vi "Pump.vi"(2 "error in (no error)":errorcluster, 3 "Pump Frequency":i32=100, 4 "Pump Cycles":i32, 5 "LINX Resource":T1={"IO"=enum."Remote", "Interface"=enum."Serial", "LINX Device Config"={"Interface"=enum."Serial", "COM Port"="COM13", "TCP Configuration"={"IP Address"="", "Port"=0}, "Device Family"=1, "Device ID"=1, "Device Name"="myRIO-1900", "TCP Ref"=refnum, "Channels"={"DI"=[0, 1, 2, 3, 4, 5, 6, 7, 8, 9, 10, 11, 12, 13, 14, 15, 16, 17, 18, 19, 20, 21, 22, 23, 24, 25, 26, 27, 28, 29, 30, 31, 32, 33, 34, 35, 36, 37, 38, 39, 40, 41, 42, 43, 44, 45, 46], "DO"=[0, 1, 2, 3, 4, 5, 6, 7, 8, 9, 10, 11, 12, 13, 14, 15, 16, 17, 18, 19, 20, 21, 22, 23, 24, 25, 26, 27, 28, 29, 30, 31, 32, 33, 34, 35, 36, 37, 38, 39, 40, 41, 42, 43, 44, 45, 46], "AI"=[0, 1, 2, 3, 4, 5, 6, 7, 8, 9, 10, 11], "AO"=[], "PWM"=[3, 5, 6, 9, 10], "QE"=[], "UART"=[0, 1], "I2C 2"=[0], "SPI"=[0], "CAN"=[], "Servo"=[], "AI Ref (V)"=0.0, "AI Resolution (Bits)"=0, "AO Ref (V)"=0.0, "AO Resolution (Bits)"=0}}}) -> (0 "error out":errorcluster, 1 "LINX Resource out":T1)   [LabVIEW 2018]
uses:
  <vilib>/MakerHub/LINX/Private/Type Defs/LINX Ref.ctl
  <vilib>/MakerHub/LINX/Private/Type Defs/Platform.ctl
  <vilib>/MakerHub/LINX/Private/Type Defs/Interface.ctl
  <vilib>/MakerHub/LINX/Private/Device/Type Defs/LINX Device Config.ctl
  <vilib>/MakerHub/LINX/Private/Device/Type Defs/TCP Config.ctl
  <vilib>/MakerHub/LINX/Private/Device/Type Defs/Channels.ctl
  <vilib>/MakerHub/LINX/Public/Peripherals/Digital/Digital Write N Chans.vi
  <vilib>/MakerHub/LINX/Private/Local IO/LinxDigitalWrite.vi
  <vilib>/MakerHub/LINX/Public/Utilities/Check Channel.vi
  <vilib>/MakerHub/LINX/Private/Utilties/Generate Error.vi
  <vilib>/MakerHub/LINX/LMH-LINX.lvlib
  <vilib>/MakerHub/LINX/Private/Device/Device.lvlib
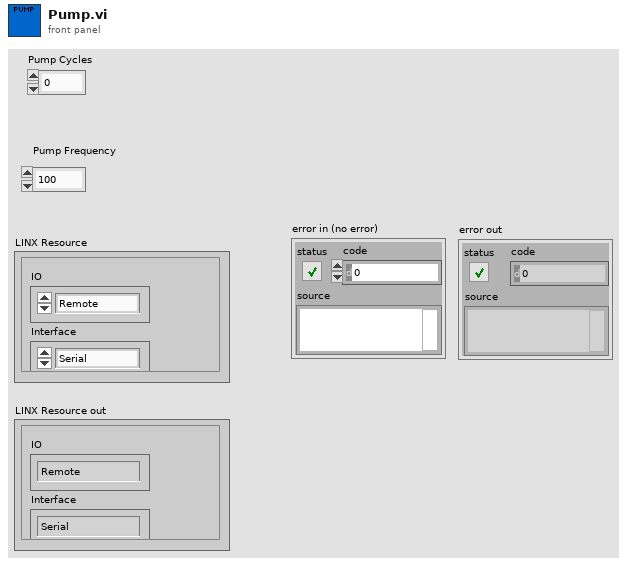
[diagram p1: front panel]
types:
  T1 = typedef "LMH-LINX.lvlib/LINX Ref.ctl" = cluster{"IO":T2, "Interface":T3, "LINX Device Config":T4}
  T2 = typedef "LMH-LINX.lvlib/Platform.ctl" = enum16{"Remote", "Local"}
  T3 = typedef "LMH-LINX.lvlib/Interface.ctl" = enum16{"Serial", "TCP"}
  T4 = typedef "LMH-LINX.lvlib/Device.lvlib/LINX Device Config.ctl" = cluster{"Interface":T3, "COM Port":refnum<visa-resource-name>, "TCP Configuration":T5, "Device Family":u8, "Device ID":u8, "Device Name":string, "TCP Ref":refnum<k5>, "Channels":T6}
  T5 = typedef "LMH-LINX.lvlib/Device.lvlib/TCP Config.ctl" = cluster{"IP Address":string, "Port":u16}
  T6 = typedef "LMH-LINX.lvlib/Channels.ctl" = cluster{"DI":u8[], "DO":u8[], "AI":u8[], "AO":u8[], "PWM":u8[], "QE":u8[], "UART":u8[], "I2C 2":u8[], "SPI":u8[], "CAN":u8[], "Servo":u8[], "AI Ref (V)":dbl, "AI Resolution (Bits)":u8, "AO Ref (V)":dbl, "AO Resolution (Bits)":u8}
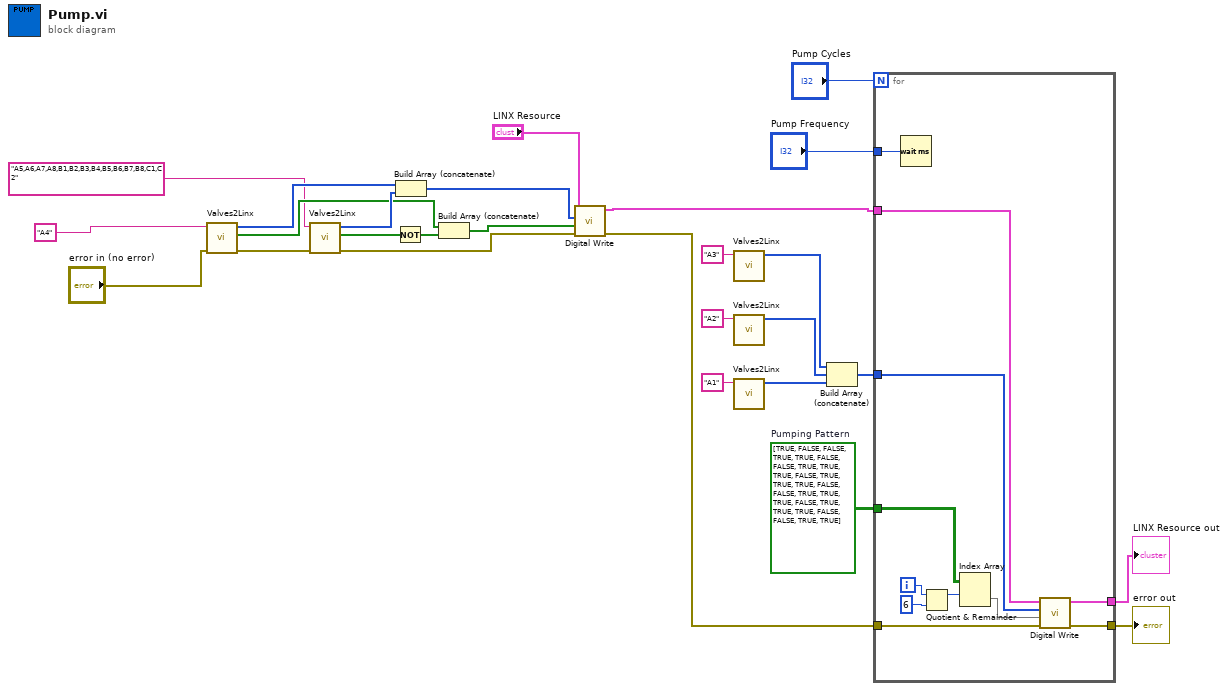
[diagram p0: block diagram]
diagram:
  w18 = bool[][] [[TRUE, FALSE, FALSE], [TRUE, TRUE, FALSE], [FALSE, TRUE, TRUE], [TRUE, FALSE, TRUE], [TRUE, TRUE, FALSE], [FALSE, TRUE, TRUE], [TRUE, FALSE, TRUE], [TRUE, TRUE, FALSE], [FALSE, TRUE, TRUE]]  # Pumping Pattern
  n1 = call "Valves2Linx.vi"("error in (no error)"="error in (no error)", "Valve (A1-C8),\n comma separated"="A4") -> ("error out"=w10:errorcluster, "Array"=w12:bool[], "Array 2"=w13:i32[])  [unwired: 7 in]
  n2 = call "Valves2Linx.vi"("error in (no error)"=w10, "Valve (A1-C8),\n comma separated"="A5,A6,A7,A8,B1,B2,B3,B4,B5,B6,B7,B8,C1,C2") -> ("error out"=w6:errorcluster, "Array"=w15:bool[], "Array 2"=w14:i32[])  [unwired: 7 in]
  n3 = Not(x=w15) -> (.not. x?=w11:bool[])
  n4 = Build Array (concatenate)(w13, w14) -> (w4:i32[])
  n5 = Build Array (concatenate)(w12, w11) -> (w5:bool[])
  n6 = call-poly <vilib>:"Digital Write.vi"("Error In"=w6, "Values"=w5, "DO Channels"=w4, "LINX Resource"="LINX Resource") -> ("Error Out"=w1:errorcluster, "LINX Resource"=w2:T1)  [unwired: 6 in]
  n7 = call "Valves2Linx.vi"("Valve (A1-C8),\n comma separated"="A3") -> ("Array 2"=w22:i32[])  [unwired: 8 in, 2 out]
  n8 = call "Valves2Linx.vi"("Valve (A1-C8),\n comma separated"="A2") -> ("Array 2"=w21:i32[])  [unwired: 8 in, 2 out]
  n9 = call "Valves2Linx.vi"("Valve (A1-C8),\n comma separated"="A1") -> ("Array 2"=w20:i32[])  [unwired: 8 in, 2 out]
  n10 = Build Array (concatenate)(w22, w21, w20) -> (w19:i32[])
  n11 = for {
    N: "Pump Cycles" -> [_]
    tunnel: "Pump Frequency" -> [w38]
    tunnel: w1 -> [w28]
    tunnel: w2 -> [w29]
    tunnel: w19 -> [w30]
    tunnel: w18 -> [w31]
    tunnel: [w33] -> w17
    tunnel: [w34] -> w16
    i -> [w32]
    n12 = Wait (ms)(milliseconds to wait=w38) -> ()  [unwired: 1 out]
    n13 = Quotient & Remainder(x=w32, y=6) -> (x-y*floor(x/y)=w37:i32)  [unwired: 1 out]
    n14 = Index Array(array=w31, index (row)=w37) -> (element=w36:bool[])  [unwired: 1 in]
    n15 = call-poly <vilib>:"Digital Write.vi"("Error In"=w28, "Values"=w36, "DO Channels"=w30, "LINX Resource"=w29) -> ("Error Out"=w34:errorcluster, "LINX Resource"=w33:T1)  [unwired: 6 in]
  }
  "error out" <- w16
  "LINX Resource out" <- w17
